vi "Constants.vi"() -> ()   [LabVIEW 2017]
panel:
  in  "Turn Travel\nUnits Per Rotation":dbl=3600.0
  in  "Rotations\nTo Travel":dbl=6.0
  in  "Motion Profile Gains":T1={"kP"=1.0, "kI "=0.0, "kD"=0.0, "kF"=0.1504411764705882, "I Zone"=400.0, "Peak Out"=1.0}
  in  "Velocity Gains":T1={"kP"=0.1, "kI "=0.0, "kD"=20.0, "kF"=0.1504411764705882, "I Zone"=300.0, "Peak Out"=0.5}
  in  "Turn Gains":T1={"kP"=2.0, "kI "=0.0, "kD"=4.0, "kF"=0.0, "I Zone"=200.0, "Peak Out"=1.0}
  in  "Distance Gains":T1={"kP"=0.1, "kI "=0.0, "kD"=0.0, "kF"=0.0, "I Zone"=100.0, "Peak Out"=0.5}
  in  "Neutral\nDeadband":dbl=0.001
  in  "Base Trajectory\nPeriod Ms":i32
  in  "Timeout Ms":i32=10
  in  "Pigeon Units\nPer Rotatoin":i32=8192
  in  "Encoder Units\nPer Rotation":i32=51711
  in  "Heading Sensor\nChoice":i32
  in  "Sensor Units\nPer Rotation":i32=4096
  in  "Number of \nButtons plus one":i32=10
  in  "Motion Profile Slot":i32=3
  in  "Velocity Slot":i32=2
  in  "Turn Slot":i32=1
  in  "Distance Slot":i32
  in  "PID Turn":i32=1
  in  "PID Primary":i32
  in  "REMOTE 1":i32=1
  in  "REMOTE 0":i32
  # "How many\nbuttons to poll:\n10 means [1,9]\nare polled"
  # "How many\nsensor units\nper rotation:\nCTRE Mag\nEncoder"
  # "How to measure\nrobot heading:\n0 - Diff b/w left & right\n1 - Pigeon IMU"
  # "Empirically\nmeasure the\ndifference\nbetween \nencoders per\n360 degrees"
  # "Scales units to\n3600 per rotation.\nThis is nice, as it\nmeans one unit is\n0.1 degrees."
  # "Property of pigeon\nshould not be\nchanged"
  # "Constants"
  # "You shouldn't need\nto change these"
  # "0 - Skip confirmation\nNonZero - Wait and log\nto DS if something fails"
  # "Base Period\nto add to each\npoint's unique\nDurattion"
  # "Motor's\nNeutral deadband"
  # "0.1504411764705882 = 1023/6800"
  # "1023 = Max Output\n6800 = Measured Max Output"
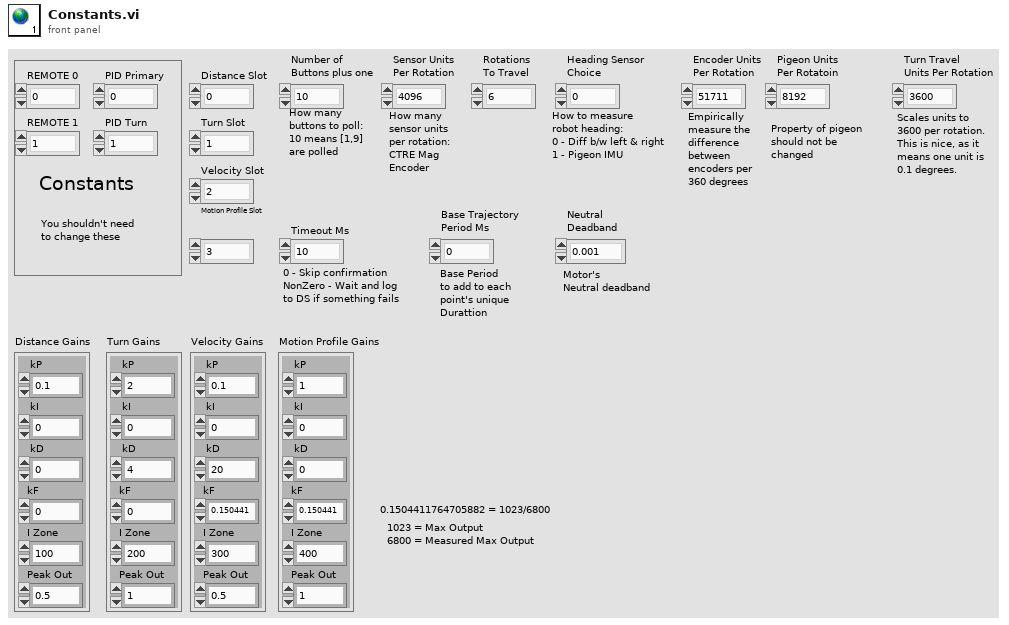
[diagram p1: front panel]
types:
  T1 = cluster{"kP":dbl, "kI ":dbl, "kD":dbl, "kF":dbl, "I Zone":dbl, "Peak Out":dbl}
diagram:
